vi "Tilt alarm.vi"(0 "X-Array-Shift-in":dbl[](array[numeric]), 1 "Y-Array-Shift-in":dbl[](array[numeric]), 3 "X-Stored-Shift-in":dbl, 4 "Y-Stored-Shift-in":dbl, 5 "Grounded?":bool, 6 "error in (no error)":errorcluster, 7 "Iterations":dbl, 8 "Filter?":bool, 9 "Accelerometer Ref X in":T1, 12 "Radius":dbl=5.0, 13 "Accelerometer Ref Y In":T1, 14 "high cutoff freq: fh":dbl=50.0) -> (20 "X-Array-Shift-out":dbl[](array[numeric]), 21 "Y-Array-Shift-out":dbl[](array[numeric]), 23 "X-Stored-Shift-out":dbl, 24 "Y-Stored-Shift-out":dbl, 25 "Alarm":bool, 26 "error out":errorcluster)   [LabVIEW 2018]
uses:
  <vilib>/myRIO/Instrument Drivers/Onboard Devices/Accelerometer/typedefs/Accelerometer Reference.ctl
  <vilib>/myRIO/Common/Instrument Driver Framework/Utilities/typedefs/myRIO Generic Hardware Reference.ctl
  <vilib>/myRIO/Common/Instrument Driver Framework/Utilities/typedefs/Hardware Version Enum.ctl
  <vilib>/myRIO/Common/Instrument Driver Framework/Utilities/typedefs/myRIO v1.0 Reference.ctl
  <vilib>/myRIO/Common/Instrument Driver Framework/Utilities/typedefs/Generic FPGA Reference.ctl
  <vilib>/myRIO/Common/Instrument Driver Framework/myRIO v1.0/Accelerometer/typedefs/Accelerometer Channels List.ctl
  <vilib>/myRIO/Common/Instrument Driver Framework/myRIO v1.0/Accelerometer/typedefs/Accelerometer Channels Enum.ctl
  <vilib>/Analysis/3filter.llb/Filter Passband Type.ctl
  <vilib>/Utility/error.llb/Error Cluster From Error Code.vi
  <vilib>/myRIO/Common/Instrument Driver Framework/myRIO v1.0/Accelerometer/vis/myRIO v1.0 Read Accelerometer.vi
  <vilib>/Analysis/3filter.llb/Butterworth Filter (DBL).vi
  <vilib>/myRIO/Instrument Drivers/Onboard Devices/Accelerometer/Accelerometer.lvlib
  <vilib>/Analysis/NI_AALBase.lvlib
panel:
  out "X-Actual":dbl
  out "Y-Actual":dbl
  out "Y-Stored":dbl
  out "X-Stored":dbl
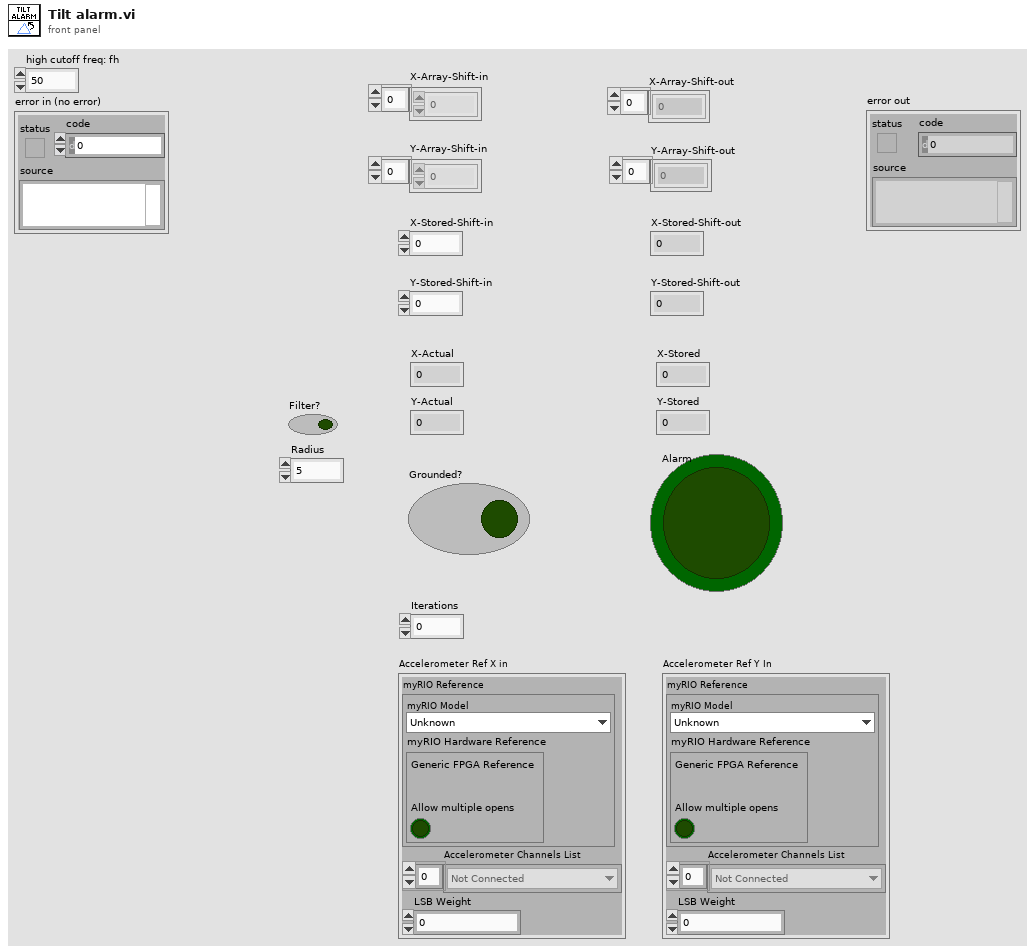
[diagram p1: front panel]
types:
  T1 = typedef "Accelerometer.lvlib/Accelerometer Reference.ctl" = cluster{"myRIO Reference":T2, "Accelerometer Channels List":T6, "LSB Weight":dbl}
  T2 = typedef "myRIO Generic Hardware Reference.ctl" = cluster{"myRIO Model":T3, "myRIO Hardware Reference":T4}
  T3 = typedef "Hardware Version Enum.ctl" = enum16{"Unknown", "myRIO-1900", "myRIO-1950", "roboRIO", "NI ELVIS RIO CM", "ELVIS III"}
  T4 = typedef "myRIO v1.0 Reference.ctl" = cluster{"Generic FPGA Reference":T5, "Allow multiple opens":bool}
  T5 = typedef "Generic FPGA Reference.ctl" = refnum<k20>
  T6 = typedef "Accelerometer Channels List.ctl" = T7[]
  T7 = typedef "Accelerometer Channels Enum.ctl" = enum16{"Not Connected", "X-Axis", "Y-Axis", "Z-Axis"}
  T8 = typedef "NI_AALBase.lvlib/Filter Passband Type.ctl" = enum32{"Lowpass", "Highpass", "Bandpass", "Bandstop"}
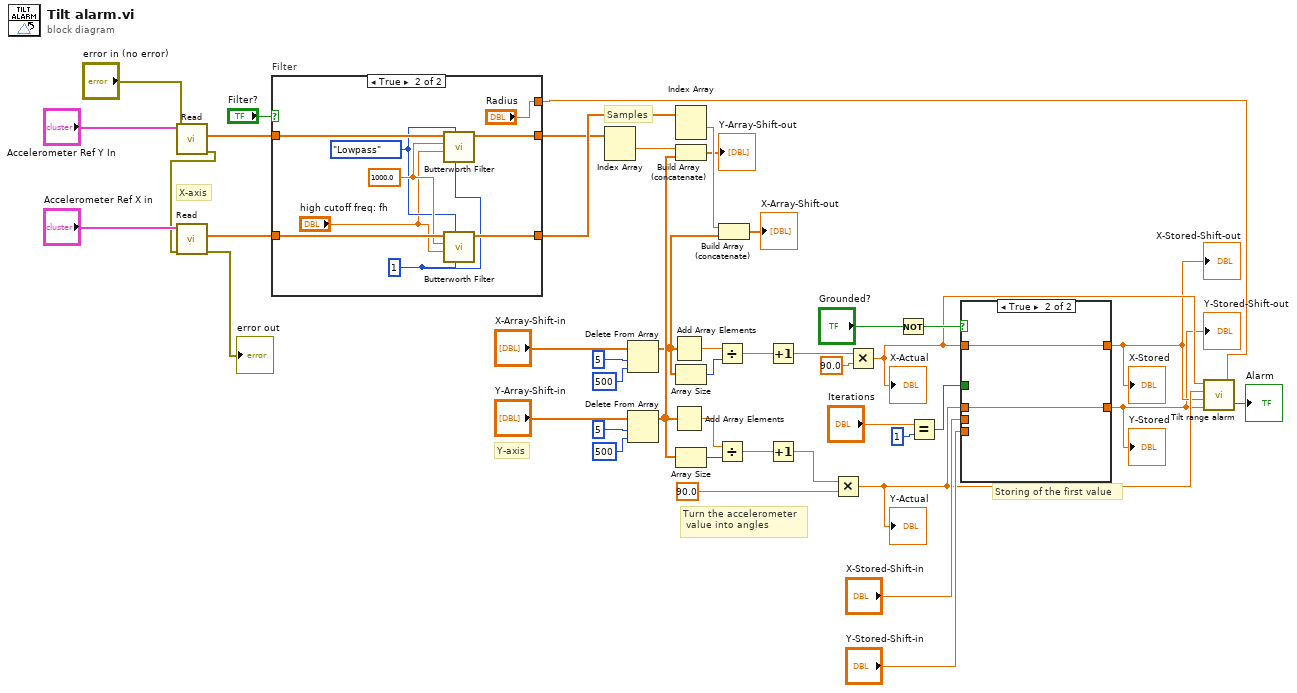
[diagram p0: block diagram]
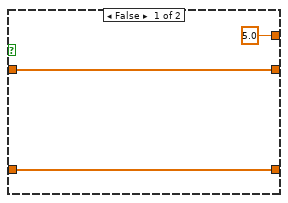
[diagram p2: hidden frame]
diagram:
  # "Storing of the first value"
  # "Turn the accelerometer\n value into angles"
  # "Samples"
  # "Y-axis"
  # "X-axis"
  n1 = call <vilib>:"Read.vi"("error in (no error)"="error in (no error)", "Accelerometer Ref In"="Accelerometer Ref Y In") -> ("error out"=w2:errorcluster, "Values"=w7:dbl[])  [unwired: 7 in, 1 out]
  n2 = call <vilib>:"Read.vi"("error in (no error)"=w2, "Accelerometer Ref In"="Accelerometer Ref X in") -> ("error out"=→"error out":errorcluster, "Values"=w9:dbl[])  [unwired: 7 in, 1 out]
  n3 = case "Filter" shown="True" "Filter?" {
    tunnel: w9 -> [w48 w57]
    tunnel: [w48 w56] -> w8
    tunnel: w7 -> [w47 w55]
    tunnel: [w47 w54] -> w6
    tunnel: [5.0 ("Radius") "Radius"] -> w4
    frame False {
    }
    frame True {
      w51 = 1 ("order")
      w52 = Filter_Passband_Type."Lowpass" ("filter type")
      w53 = 1000.0 ("sampling freq: fs")
      n4 = call-poly <vilib>:"Butterworth Filter.vi"("order"=w51, "filter type"=w52, "high cutoff freq: fh"="high cutoff freq: fh", "sampling freq: fs"=w53, "X"=w55) -> ("Filtered X"=w54:dbl[])  [unwired: 3 in, 1 out]
      n5 = call-poly <vilib>:"Butterworth Filter.vi"("order"=w51, "filter type"=w52, "high cutoff freq: fh"="high cutoff freq: fh", "sampling freq: fs"=w53, "X"=w57) -> ("Filtered X"=w56:dbl[])  [unwired: 3 in, 1 out]
    }
  }
  n6 = Index Array(array=w6) -> (element #1=w15:dbl)  [unwired: 2 in, 1 out]
  n7 = Delete From Array(array="X-Array-Shift-in", length=5, index=500) -> (array with subset deleted=w36:dbl[])  [unwired: 1 out]
  n8 = Delete From Array(array="Y-Array-Shift-in", length=5, index=500) -> (array with subset deleted=w38:dbl[])  [unwired: 1 out]
  n9 = Add Array Elements(numeric array=w36) -> (sum=w37:dbl)
  n10 = Add Array Elements(numeric array=w38) -> (sum=w40:dbl)
  n11 = Index Array(array=w8) -> (element #1=w45:dbl)  [unwired: 2 in, 1 out]
  n12 = Build Array (concatenate)(w15, w38) -> (→"Y-Array-Shift-out":dbl[])
  n13 = Array Size(array=w36) -> (size(s)=w35:i32)
  n14 = Array Size(array=w38) -> (size(s)=w39:i32)
  n15 = Divide(x=w37, y=w35) -> (x/y=w30:dbl)
  n16 = Divide(x=w40, y=w39) -> (x/y=w31:dbl)
  n17 = Build Array (concatenate)(w45, w36) -> (→"X-Array-Shift-out":dbl[])
  n18 = Increment(x=w30) -> (x+1=w29:dbl)
  n19 = Increment(x=w31) -> (x+1=w32:dbl)
  n20 = Multiply(x=w32, y=90.0) -> (x*y=w13:dbl)
  "Y-Actual" <- w13
  n21 = Multiply(x=w29, y=90.0) -> (x*y=w14:dbl)
  "X-Actual" <- w14
  n22 = Not(x="Grounded?") -> (.not. x?=w17:bool)
  n23 = Equal?(x="Iterations", y=1) -> (x = y?=w27:bool)
  n24 = case shown="True" w17 {
    tunnel: w14 -> [w59 w70]
    tunnel: w13 -> [w58 w69]
    tunnel: [w60 w70] -> w12
    tunnel: [w62 w69] -> w11
    tunnel: "X-Stored-Shift-in" -> [w61 _]
    tunnel: "Y-Stored-Shift-in" -> [w63 _]
    tunnel: w27 -> [w64 _]
    frame False {
      n25 = case shown="True" w64 {
        tunnel: w63 -> [w66 _]
        tunnel: [w66 w67] -> w62
        tunnel: w61 -> [w65 _]
        tunnel: [w65 w68] -> w60
        tunnel: w59 -> [_ w68]
        tunnel: w58 -> [_ w67]
        frame False {
        }
        frame True {
        }
      }
    }
    frame True {
    }
  }
  "X-Stored-Shift-out" <- w12
  "Y-Stored-Shift-out" <- w11
  "X-Stored" <- w12
  "Y-Stored" <- w11
  n26 = call "Tilt range alarm.vi"("Radius"=w4, "Y-Stored"=w11, "X-Stored"=w12, "Y-Actual"=w13, "X-Actual"=w14) -> ("Alarm"=→"Alarm":bool)
